vi "Send Stop Command To Robot.vi"(8 "error in (no error)":errorcluster) -> (0 "error out":errorcluster)   [LabVIEW 2016]
uses:
  Communication Global variables.vi
  <vilib>/addons/_JKI.lib/REST Client/classes/REST Client/REST Client.lvclass
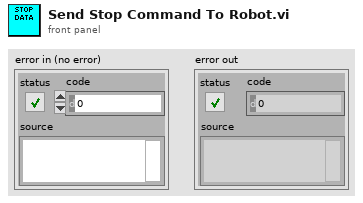
[diagram p1: front panel]
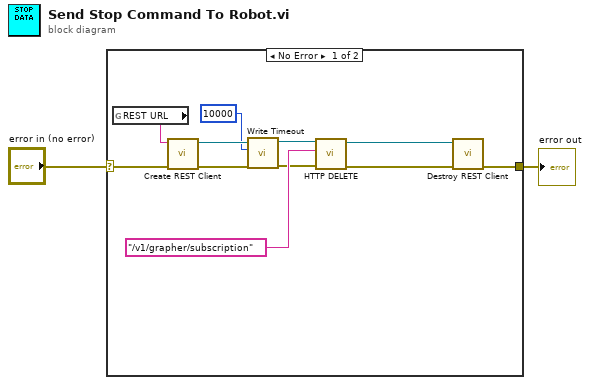
[diagram p0: block diagram]
diagram:
  n1 = case shown="No Error" "error in (no error)" {
    selector: "error in (no error)" -> [w13 w14]
    tunnel: [w8 w14] -> w1
    frame No Error {
      n2 = global read "Communication Global variables.vi" "REST URL"() -> (w10:string)
      n3 = call <vilib>:"Create REST Client.vi"("error in (no error)"=w13, "Base URL"=w10) -> ("error out"=w7:errorcluster, "REST Client out"=w5:refnum<class "REST Client.lvclass">)  [unwired: 8 in]
      n4 = call-dynamic "Write Timeout.vi"("error in (no error)"=w7, "Timeout"=10000, "REST Client in"=w5) -> ("error out"=w6:errorcluster, "REST Client out"=w4:refnum<class "REST Client.lvclass">)  [unwired: 7 in]
      n5 = call-dynamic "HTTP DELETE.vi"("error in (no error)"=w6, "Path"="/v1/grapher/subscription", "REST Client in"=w4) -> ("error out"=w9:errorcluster, "REST Client out"=w11:refnum<class "REST Client.lvclass">)  [unwired: 3 in, 4 out]
      n6 = call-dynamic "Destroy REST Client.vi"("error in (no error)"=w9, "REST Client in"=w11) -> ("error out"=w8:errorcluster)  [unwired: 9 in]
    }
    frame Error {
    }
  }
  "error out" <- w1
